vi "Launcher.vi"   [LabVIEW 2020]
uses:
  Businness Logic/Businness Logic/Businness Logic.lvclass
  <vilib>/ActorFramework/Actor/Actor.lvclass
  C:/Program Files (x86)/National Instruments/LabVIEW 2020/vi.lib/ActorFramework/Actor/Actor.lvclass
  D:/Storage/Source Code/Clase AF/ClaseAF/08 Acquisition AF/Businness Logic/Businness Logic/Businness Logic.lvclass
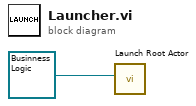
[diagram p0: block diagram]
diagram:
  n1 = call <vilib>:"Launch Root Actor.vi"("Actor"=refnum<class "Businness Logic.lvclass"> refnum ("Businness Logic.lvlib:Businness Logic.lvclass")) -> ()  [unwired: 9 in, 2 out]
